vi "Configure StopVelocity Core.vi"(8 "error in (no error)":errorcluster, 9 "StopVelocity":dbl, 10 "AxisNumber":u8, 11 "CS++Nanotec in":refnum<class "CS++Nanotec.lvclass">) -> (0 "error out":errorcluster, 3 "CS++Nanotec out":refnum<class "CS++Nanotec.lvclass">)   [LabVIEW 2015, in "CS++Nanotec.lvlib" / "CS++Nanotec.lvclass"]
doc: "Configures the stop (maximum) velocity of the axis."
uses:
  CS++Nanotec.lvclass
  CS++Nanotec.lvclass/CS++Nanotec.ctl
  instr.lib/NanotecSMCPD/NanotecSMCPDDriver.lvlib
  CSPP_DeviceBase/CS++Motor/CS++Motor.lvclass
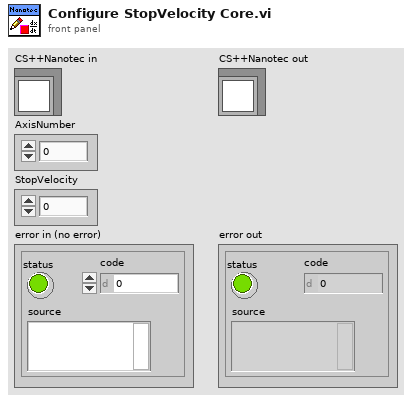
[diagram p1: front panel]
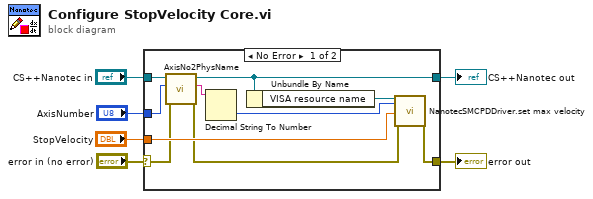
[diagram p0: block diagram]
diagram:
  n1 = case shown="No Error" "error in (no error)" {
    selector: "error in (no error)" -> [w10 w17]
    tunnel: [w16 w17] -> w5
    tunnel: "CS++Nanotec in" -> [w12 w18]
    tunnel: "AxisNumber" -> [w8 _]
    tunnel: "StopVelocity" -> [w14 _]
    tunnel: [w11 w18] -> w1
    frame No Error {
      n2 = call "AxisNo2PhysName.vi"("error in (no error)"=w10, "AxisNumber"=w8, "CS++Motor in"=w12) -> ("error out"=w9:errorcluster, "PhysicalChannelName"=w13:string, "CS++Motor out"=w11:refnum<class "CS++Nanotec.lvclass">)  [unwired: 6 in]
      n3 = Decimal String To Number(string=w13) -> (number=w7:i32)  [unwired: 2 in, 1 out]
      n4 = Unbundle By Name(w11) -> ("VISA resource name"=w15:refnum<visa-resource-name>)
      n5 = call "NanotecSMCPDDriver.set max velocity.vi"("VISA resource name"=w15, "contollerID"=w7, "maxVelocity [Hz]"=w14, "error in (no error)"=w9) -> ("error out"=w16:errorcluster)  [unwired: 13 in, 2 out]
    }
    frame Error {
    }
  }
  "error out" <- w5
  "CS++Nanotec out" <- w1
